vi "MIN_BPM.vi"() -> (3 "MIN_BPM":i32=8)   [LabVIEW 2018]
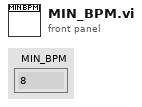
[diagram p1: front panel]
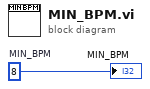
[diagram p0: block diagram]
diagram:
  w1 = 8  # MIN_BPM
  "MIN_BPM" <- w1
